vi "BNC555.constructor.vi"(0 "name":string, 2 "data in":string, 5 "error in(no error)":errorcluster) -> (14 "i ref out":refnum<vi>, 16 "data out":string, 19 "error out":errorcluster)   [LabVIEW 2014, in "BNC555.lvlib"]
doc: "Berkeley Nucleonics Delay Generator 555.\n\nauthor: Holger Brand, GSI\n\nLicense Agreement for this software:\n\nCopyright (C)\nGesellschaft für Schwerionenforschung, GSI\nPlanckstr. 1\n64291 Darmstadt\nGermany\n\nContact: D.Beck@gsi.de \n\nThis program is free software; you can redistribute it and/or modify it under the terms of the \nGNU General Public License as published by the Free Software Foundation; either version 2 of \nthe license, or (at your option) any later version.\n\nThis program is distributed in the hope that it will be useful, but WITHOUT ANY WARRANTY; \nwithout even the implied warranty of MERCHANTABILITY or FITNESS FOR A PARTICULAR PURPOSE. See the GNU General License for more details (http://www.gnu.org).\n\nGesellschaft für Schwerionenforschung, GSI\nPlanckstr. 1, 64291 Darmstadt, Germany\nFor all questions and ideas contact: M.Richter@gsi.de, H.Brand@gsi.de or D.Beck@gsi.de.\nLast update: 16-JUN-2004"
uses:
  BNC555.lvlib
  CS_PHELIX/PH_Basics/PH_PSDBWriter/PH_PSDBWriter.lvlib
  CS_PHELIX/PH_Basics/PH_Class/PH_Class.lvlib
  CS_PHELIX/PH_Basics/PH_StatusHandler/PH_StatusHandler.lvlib
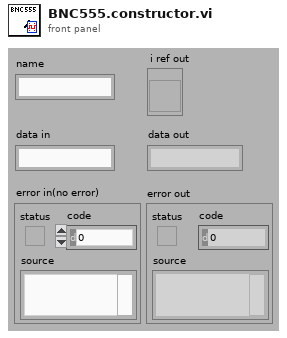
[diagram p1: front panel]
types:
  T1 = enum16{"All Info", "State", "Period", "Oscillator", "Mode", "Trigger"}
  T2 = enum16{"SetAttribute", "GetAttribute", "CreateAttribute", "DestroyAttribute", "DestroyAllAtributes"}
  T3 = enum16{"All Info", "State (On/Off)", "Output Config", "Mode Config", "Pulse Config", "Gate Config"}
  T4 = typedef "BNC555.lvlib/BNC555.i attribute.ctl" = cluster{"Information":cluster{"VISA resource name":refnum<visa-resource-name>, "Baud Rate (1:9600)":u16}, "Channel Array":T5[], "System":T6, "GUI Refs":cluster{"Delete":refnum<vi>, "Information":refnum<vi>, "System":refnum<vi>, "Channel Array":refnum<vi>, "Device Error":refnum<vi>, "Instr Driver Revision":refnum<vi>, "Instr Firmware Revision":refnum<vi>, "Instr Option":refnum<vi>, "Self-Test Response":refnum<vi>}, "Service IDs Channelinfo":i32[], "Service ID T0 Mode":i32}
  T5 = typedef "BNC555 - Driver np.lvlib/BNC555 All Chan Parameters.ctl" = cluster{"Chan #":i32, "Chan State":bool, "Chan Delay":dbl, "Chan Width":dbl, "Chan Mode":enum16{"Normal", "Single", "Burst", "Divide by N"}, "Chan Burst #":u32, "Chan Divide #":u32, "Chan Pol Out":enum16{"Normal", "Complement", "Inverted"}, "Chan Level Out":enum16{"TTL", "Adjustable", "35 Volt"}, "Chan Lev Adjust":dbl, "Chan Gate Pol":enum16{"Normal", "Complement", "Inverted"}, "Chan Gate State":bool}
  T6 = typedef "BNC555 - Driver np.lvlib/BNC555 All Sys Parameters.ctl" = cluster{"Sys Period":dbl, "Sys Oscillator":bool, "Sys Mode":enum16{"Normal", "Single", "Burst", "Duty Cycle"}, "Sys Burst #":u32, "Sys DC On":u32, "Sys DC Off":u32, "Sys Trig Mode":enum16{"Disabled", "Triggered", "Gated"}, "Sys Trig Lev":dbl, "Sys Gate State":bool, "Sys Trig Edge":bool, "Sys State":bool}
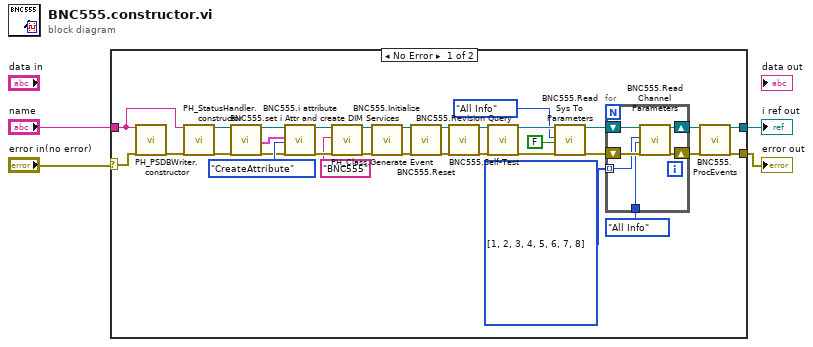
[diagram p0: block diagram]
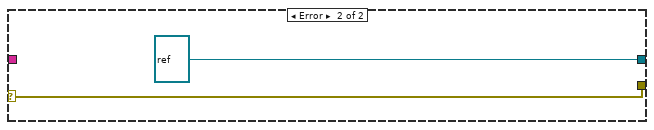
[diagram p2: hidden frame]
diagram:
  n1 = case shown="No Error" "error in(no error)" {
    selector: "error in(no error)" -> [w17 w43]
    tunnel: "name" -> [w13 _]
    tunnel: [w7 refnum<vi> refnum ("i ref out")] -> w3
    tunnel: [w5 w43] -> w2
    frame No Error {
      w34 = i32[] [1, 2, 3, 4, 5, 6, 7, 8] items=["System (To)", "Channel A", "Channel B", "Channel C", "Channel D", "Channel E", "Channel F", "Channel G", "Channel H"]
      n2 = call "PH_PSDBWriter.constructor.vi"("name"=w13, "error in"=w17) -> ("error out"=w20:errorcluster)  [unwired: 15 in, 2 out]
      n3 = call "PH_StatusHandler.constructor.vi"("name"=w13, "error in(no error)"=w20) -> ("i ref out"=w14:refnum<vi>, "error out"=w15:errorcluster)  [unwired: 15 in, 1 out]
      n4 = call "BNC555.set i Attr and create DIM Services.vi"("i ref in"=w14, "error in (no error)"=w15) -> ("i ref out"=w18:refnum<vi>, "i Attributes"=w16:T4, "error out"=w19:errorcluster)  [unwired: 15 in]
      n5 = call "BNC555.i attribute.vi"("VI Refnum"=w18, "CLASS.i attribute"=w16, "Action"=T2."CreateAttribute", "error in (no error)"=w19) -> ("VI Refnum out"=w23:refnum<vi>, "error out"=w22:errorcluster)  [unwired: 13 in, 1 out]
      n6 = call "PH_Class.Generate Event.vi"("i ref in"=w23, "Class"="BNC555", "error in (no error)"=w22) -> ("i ref out"=w12:refnum<vi>, "error out"=w11:errorcluster)  [unwired: 15 in]
      n7 = call "BNC555.Initialize.vi"("i ref in"=w12, "error in (no error)"=w11) -> ("i ref out"=w31:refnum<vi>, "error out"=w29:errorcluster)  [unwired: 16 in]
      n8 = call "BNC555.Reset.vi"("i ref in"=w31, "error IO"=w29) -> ("i ref out"=w32:refnum<vi>, "error out"=w27:errorcluster)  [unwired: 16 in]
      n9 = call "BNC555.Revision Query.vi"("i ref in"=w32, "error IO"=w27) -> ("i ref out"=w33:refnum<vi>, "error out"=w26:errorcluster)  [unwired: 16 in]
      n10 = call "BNC555.Self-Test.vi"("i ref in"=w33, "error IO"=w26) -> ("i ref out"=w30:refnum<vi>, "error out"=w28:errorcluster)  [unwired: 16 in]
      n11 = call "BNC555.Read Sys To Parameters.vi"("i ref in"=w30, "Parameter"=T1."All Info", "Sys State"=FALSE, "error in (no error)"=w28) -> ("i ref out"=w36:refnum<vi>, "error out"=w35:errorcluster)  [unwired: 14 in]
      n12 = for {
        tunnel: w34 -> [w38] mode=indexing
        shift-right: [w41] -> w8
        shift-left: w36 -> [w42]
        shift-right: [w39] -> w6
        shift-left: w35 -> [w40]
        tunnel: T3."All Info" ("Parameter") -> [w37]
        n13 = call "BNC555.Read Channel Parameters.vi"("i ref in"=w42, "Channel (1: Chan A)"=w38, "Parameter"=w37, "error in (no error)"=w40) -> ("i ref out"=w41:refnum<vi>, "error out"=w39:errorcluster)  [unwired: 14 in]
      }
      n14 = call "BNC555.ProcEvents.vi"("i ref in"=w8, "error in"=w6) -> ("i ref out"=w7:refnum<vi>, "error out"=w5:errorcluster)  [unwired: 16 in]
    }
    frame Error {
    }
  }
  "i ref out" <- w3
  "error out" <- w2
